vi "set_plot_scale.vi"(7 "pos_neg_both":i32=2, 8 "offset":dbl, 9 "step":dbl=10.0, 10 "round":bool=TRUE, 11 "plot_data":cluster{"array type (2D Dbl)":dbl[], dbl[]}) -> (2 "y_min":dbl, 3 "y_max":dbl)   [LabVIEW 2025]
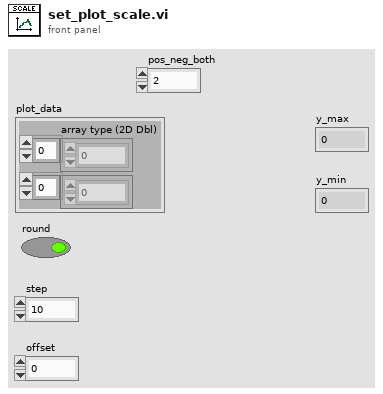
[diagram p1: front panel]
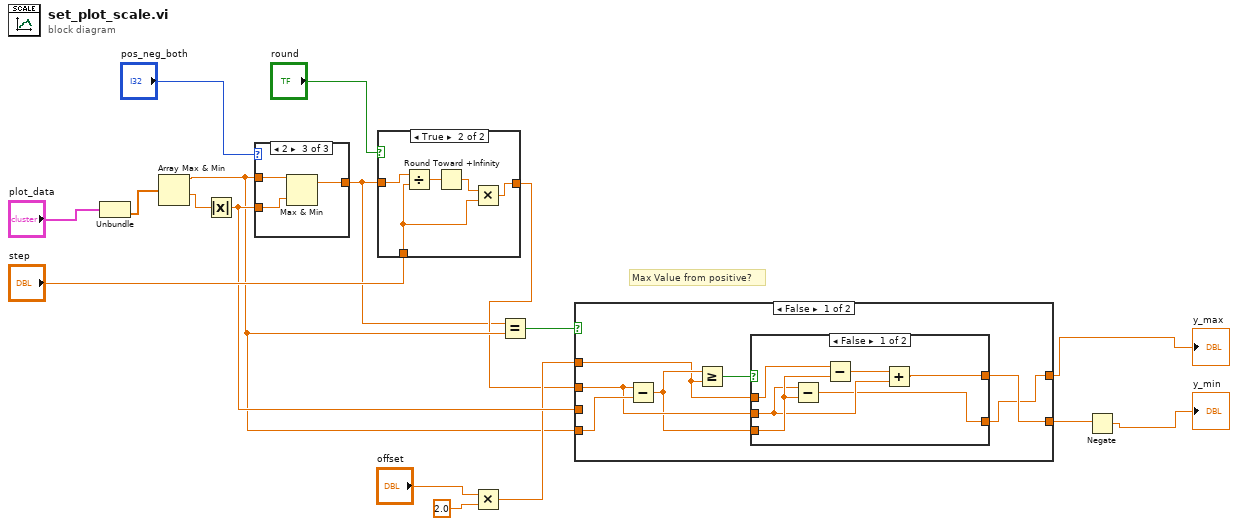
[diagram p0: block diagram]
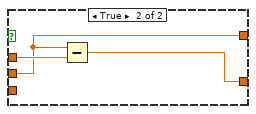
[diagram p2: hidden frame]
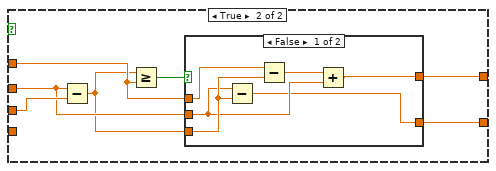
[diagram p3: hidden frame]
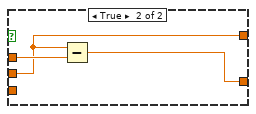
[diagram p4: hidden frame]
diagram:
  # "Max Value from positive?"
  n1 = Unbundle("plot_data") -> (w17:dbl[])  [unwired: 1 out]
  n2 = Array Max & Min(array=w17) -> (max value=w6:dbl, min value=w15:dbl)  [unwired: 2 out]
  n3 = Absolute Value(x=w15) -> (abs(x)=w8:dbl)
  n4 = case shown="2" "pos_neg_both" {
    tunnel: [w18 w19 w22] -> w1
    tunnel: w8 -> [_ w19 w21]
    tunnel: w6 -> [w18 _ w20]
    frame 0, Default {
    }
    frame 1 {
    }
    frame 2 {
      n5 = Max & Min(x=w20, y=w21) -> (max(x,y)=w22:dbl)  [unwired: 1 out]
    }
  }
  n6 = case shown="True" "round" {
    tunnel: [w23 w28] -> w2
    tunnel: w1 -> [w23 w27]
    tunnel: "step" -> [_ w24]
    frame False {
    }
    frame True {
      n7 = Divide(x=w27, y=w24) -> (x/y=w26:dbl)
      n8 = Round Toward +Infinity(x=w26) -> (ceil(x): smallest int >= x=w25:dbl)
      n9 = Multiply(x=w25, y=w24) -> (x*y=w28:dbl)
    }
  }
  n10 = Multiply(x="offset", y=2.0) -> (x*y=w7:dbl)
  n11 = Equal?(x=w1, y=w6) -> (x = y?=w10:bool)
  n12 = case shown="False" w10 {
    tunnel: w2 -> [w33 w49]
    tunnel: w8 -> [_ w51]
    tunnel: w7 -> [w31 w48]
    tunnel: w6 -> [w35 _]
    tunnel: [w30 w47] -> w5
    tunnel: [w29 w45] -> w4
    frame False {
      n13 = Subtract(x=w33, y=w35) -> (x-y=w32:dbl)
      n14 = Greater Or Equal?(x=w32, y=w31) -> (x >= y?=w34:bool)
      n15 = case shown="False" w34 {
        tunnel: w33 -> [w38 w42]
        tunnel: w31 -> [w41 w44]
        tunnel: [w37 w43] -> w29
        tunnel: w32 -> [w40 _]
        tunnel: [w36 w42] -> w30
        frame False {
          n16 = Subtract(x=w38, y=w40) -> (x-y=w37:dbl)
          n17 = Subtract(x=w41, y=w40) -> (x-y=w39:dbl)
          n18 = Add(x=w39, y=w38) -> (x+y=w36:dbl)
        }
        frame True {
          n19 = Subtract(x=w42, y=w44) -> (x-y=w43:dbl)
        }
      }
    }
    frame True {
      n20 = Subtract(x=w49, y=w51) -> (x-y=w46:dbl)
      n21 = Greater Or Equal?(x=w46, y=w48) -> (x >= y?=w50:bool)
      n22 = case shown="False" w50 {
        tunnel: w49 -> [w54 w58]
        tunnel: w48 -> [w57 w60]
        tunnel: [w53 w59] -> w47
        tunnel: w46 -> [w56 _]
        tunnel: [w52 w58] -> w45
        frame False {
          n23 = Subtract(x=w54, y=w56) -> (x-y=w53:dbl)
          n24 = Subtract(x=w57, y=w56) -> (x-y=w55:dbl)
          n25 = Add(x=w55, y=w54) -> (x+y=w52:dbl)
        }
        frame True {
          n26 = Subtract(x=w58, y=w60) -> (x-y=w59:dbl)
        }
      }
    }
  }
  "y_max" <- w4
  n27 = Negate(x=w5) -> (-x=→"y_min":dbl)
